vi "getTemperature.vi"(6 "Channel":i32, 8 "error in (no error)":errorcluster, 11 "Instrument.TC.MNK in":refnum<class "Inst.TC.MNK.lvclass">) -> (0 "error out":errorcluster, 1 "Status":string, 2 "Temperature (mK)":dbl, 3 "Instrument.TC.MNK out":refnum<class "Inst.TC.MNK.lvclass">, 4 "Finished?":bool)   [LabVIEW 2019, in "Inst.TC.MNK.lvclass"]
uses:
  Inst.TC.MNK.lvclass
  Inst.TC/Inst.TC.lvclass
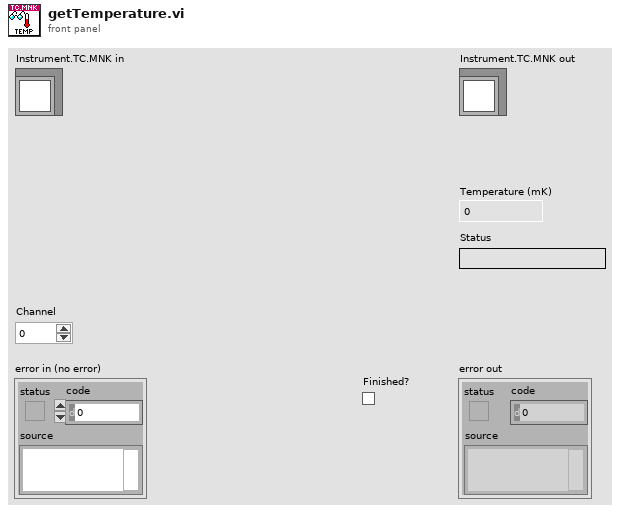
[diagram p1: front panel]
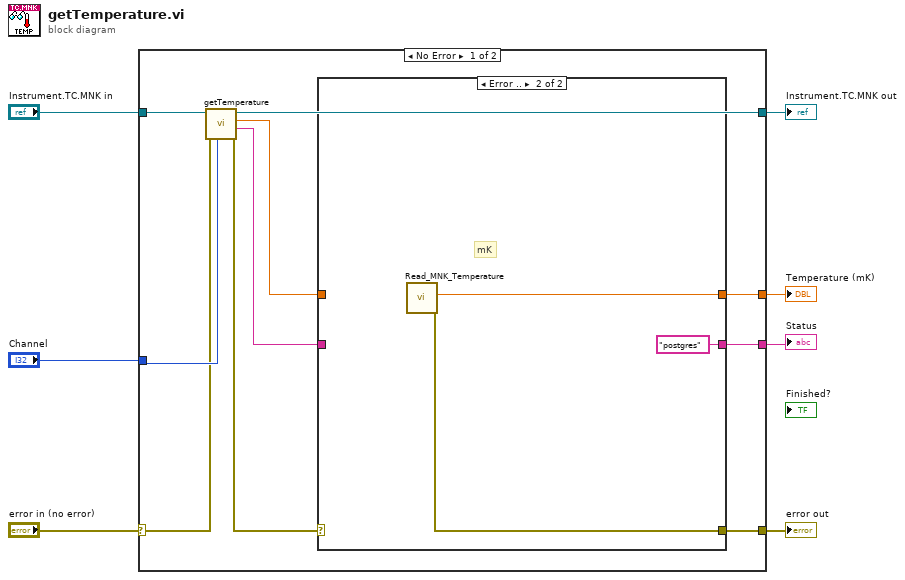
[diagram p0: block diagram]
diagram:
  n1 = case shown="No Error" "error in (no error)" {
    selector: "error in (no error)" -> [w12 w24]
    tunnel: [w17 w24] -> w6
    tunnel: [w15 w25] -> w5
    tunnel: "Instrument.TC.MNK in" -> [w14 w25]
    tunnel: [w16 _] -> w3
    tunnel: "Channel" -> [w13 _]
    tunnel: [w9 _] -> w1
    frame No Error {
      n2 = call-parent "getTemperature.vi"("Channel"=w13, "error in (no error)"=w12, "Inst.TC in"=w14) -> ("error out"=w11:errorcluster, "Status"=w8:string, "Temperature (mK)"=w10:dbl, "Inst.TC out"=w15:refnum<class "Inst.TC.MNK.lvclass">)  [unwired: 4 in, 1 out]
      n3 = case shown="Error .." w11 {
        selector: w11 -> [w18 _]
        tunnel: [w18 w22] -> w17
        tunnel: [w20 w23] -> w16
        tunnel: w10 -> [w20 _]
        tunnel: [w19 "postgres" ("Status")] -> w9
        tunnel: w8 -> [w19 _]
        frame No Error {
        }
        frame Error {
          # "mK"
          n4 = call "Read_MNK_Temperature.vi"() -> ("Error out"=w22:errorcluster, "Temperature (mK)"=w23:dbl)  [unwired: 10 in]
        }
      }
    }
    frame Error {
    }
  }
  "error out" <- w6
  "Instrument.TC.MNK out" <- w5
  "Temperature (mK)" <- w3
  "Status" <- w1
